vi "CVT1IndexReadTest.vi"() -> (3 "Unit Test Framework Results":T1)   [LabVIEW 2013, in "UnitTests.lvlib"]
uses:
  UnitTests.lvlib
  <vilib>/utf/common/utf_test_result_troll.ctl
  <vilib>/utf/common/utf_test_result.ctl
  <vilib>/utf/common/utf_test_result_failure.ctl
  <vilib>/utf/common/utf_test_comparison_operators.ctl
  <vilib>/utf/common/utf_vi_tag.ctl
  <vilib>/NI/Current Value Table/Read Index.vi
  <vilib>/NI/Current Value Table/DataTypes/I32_Read Index.vi
  <vilib>/NI/Current Value Table/Compatibility/TagConverter.vi
  <vilib>/NI/Current Value Table/Create Tags.vi
  <vilib>/NI/Current Value Table/Memory Block.vi
  <vilib>/NI/Current Value Table/DataTypes/I32_Memory Block.vi
  <vilib>/utf/NI_UnitTestFramework.lvlib
panel:
  out "Value":i32
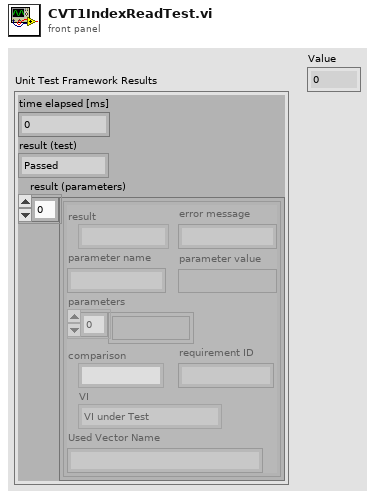
[diagram p1: front panel]
types:
  T1 = typedef "NI_UnitTestFramework.lvlib/utf_test_result_troll.ctl" = cluster{"time elapsed [ms]":u32, "result (test)":T2, "result (parameters)":T3[]}
  T2 = typedef "NI_UnitTestFramework.lvlib/utf_test_result.ctl" = enum16{"Passed", "Failed", "Error", "Skipped", "Not Processed"}
  T3 = typedef "NI_UnitTestFramework.lvlib/utf_test_result_failure.ctl" = cluster{"result":T2, "error message":string, "parameter name":string, "parameter value":variant, "parameters":variant[], "comparison":T4, "requirement ID":string, "VI":T5, "Used Vector Name":string}
  T4 = typedef "NI_UnitTestFramework.lvlib/utf_test_comparison_operators.ctl" = enum16{"=", "!=", ">", ">=", "<", "<=", "range", "symmetric tolerance", "asymmetric tolerance", "string contains", "string not contain", "array size", "string length", "array range", "by element", "array range (limit array)", "user-defined", "array contains", "array not contain", "vector length", "= (elm)", "!= (elm)", "= (case insensitive)", "!= (case insensitive)"}
  T5 = typedef "NI_UnitTestFramework.lvlib/utf_vi_tag.ctl" = enum16{"Setup VI", "VI under Test", "Teardown VI"}
  T6 = typedef "cvt_Tag Configuration.ctl" = cluster{"Name":string, "Data Type":T7, "Array":bool, "Size":u32, "Default":string, "Enum":string[], "Description":string}
  T7 = typedef "cvt_Data Types.ctl" = enum16{"Bool", "U8", "I32", "Double", "String", "Enum"}
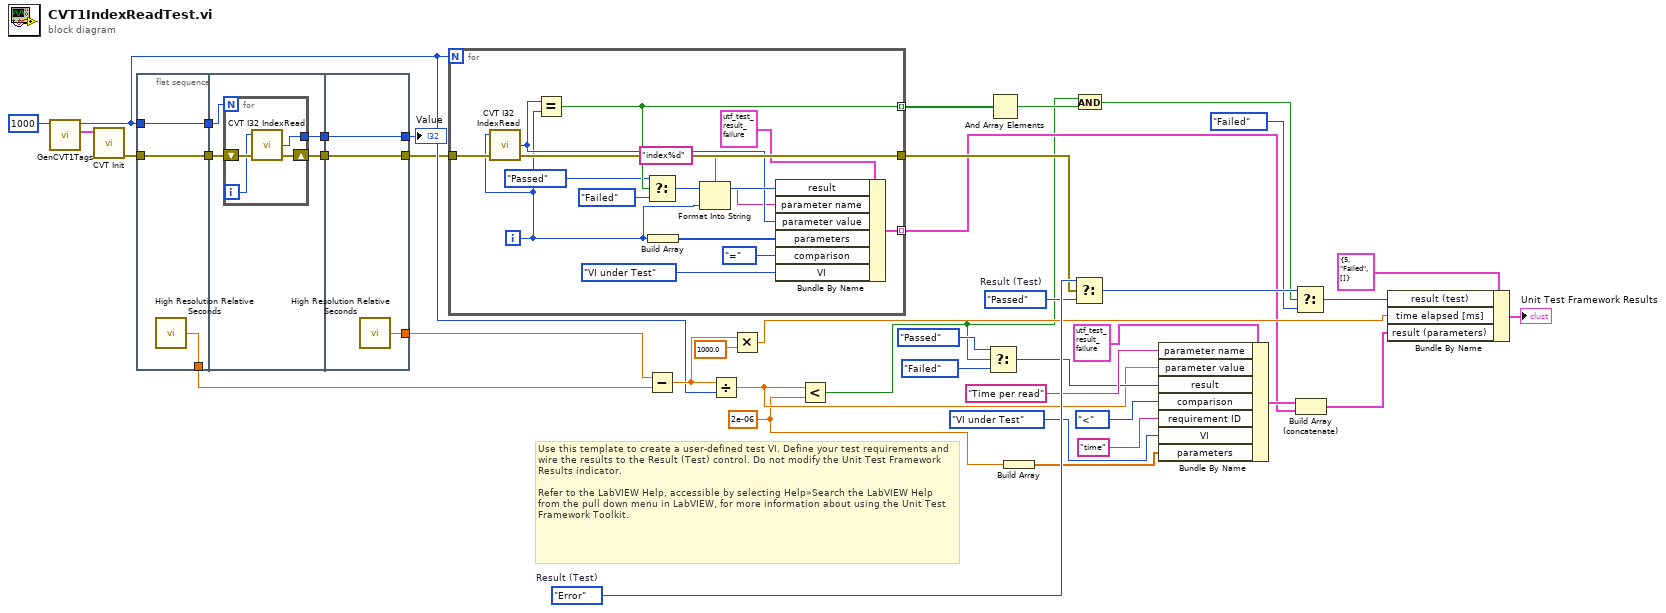
[diagram p0: block diagram]
diagram:
  w8 = 2e-06 ("y")
  w36 = utf_test_result."Error"  # Result (Test)
  w35 = utf_test_result."Passed"  # Result (Test)
  # "Use this template to create a user-defined test VI. Define your test requirements and wire the results to the Result (Test) control. Do not modify the Unit Test Framework Results indicator. \n\nRefer to the LabVIEW Help, accessible by selecting Help»Search the LabVIEW Help from the pull down menu in LabVIEW, for more information about using the Unit Test Framework Toolkit."
  n1 = call "GenCVT1Tags.vi"("Number of Tags in"=1000) -> ("Tags"=w1:T6[], "Number of Tags out"=w23:i32)  [unwired: 8 in, 1 out]
  n2 = call <vilib>:"CVT Init.vi"("Tag List"=w1) -> ("error out"=w29:errorcluster)  [unwired: 10 in]
  n3 = flat-sequence {
    tunnel: [w44] -> w38
    tunnel: w29 -> [w42]
    tunnel: [w43] -> w28
    tunnel: w23 -> [w43]
    tunnel: [w42] -> w27
    tunnel: w28 -> [w48]
    tunnel: w27 -> [w47]
    tunnel: [w46] -> w26
    tunnel: [w45] -> w3
    tunnel: [w55] -> w39
    tunnel: w26 -> [w54]
    tunnel: [w54] -> w22
    tunnel: [w53] -> w2
    tunnel: w3 -> [w53]
    frame #0 {
      n4 = call <vilib>:"High Resolution Relative Seconds.vi"() -> ("relative seconds"=w44:dbl)
    }
    frame #1 {
      n5 = for {
        N: w48 -> [_]
        shift-right: [w51] -> w46
        shift-left: w47 -> [w52]
        tunnel: [w50] -> w45
        i -> [w49]
        n6 = call <vilib>:"CVT I32 IndexRead.vi"("error in (no error)"=w52, "Tag Index"=w49) -> ("error out"=w51:errorcluster, "Value"=w50:i32)  [unwired: 2 in]
      }
    }
    frame #2 {
      n7 = call <vilib>:"High Resolution Relative Seconds.vi"() -> ("relative seconds"=w55:dbl)
    }
  }
  n8 = for {
    N: w23 -> [_]
    tunnel: w22 -> [w70]
    tunnel: [w69] -> w21
    tunnel: [w66] -> w20 mode=indexing
    tunnel: [w62] -> w6 mode=indexing
    i -> [w58]
    n9 = call <vilib>:"CVT I32 IndexRead.vi"("error in (no error)"=w70, "Tag Index"=w58) -> ("error out"=w69:errorcluster, "Value"=w59:i32)  [unwired: 2 in]
    n10 = Equal?(x=w59, y=w58) -> (x = y?=w66:bool)
    n11 = Select(t=utf_test_result."Passed" ("result"), s=w66, f=utf_test_result."Failed" ("result")) -> (s? t:f=w63:T2)
    n12 = Build Array(w58) -> (w60:i32[])
    n13 = Format Into String(format string="index%d", w58) -> (resulting string=w57:string)  [unwired: 2 in, 1 out]
    n14 = Bundle By Name(cluster=T3 {"result"=enum."Passed", "error message"="", "parameter name"="", "parameter value"=variant, "parameters"=[], "comparison"=enum."=", "requirement ID"="", "VI"=enum."Setup VI", "Used Vector Name"=""} ("Unit Test Framework - result (parameters)"), "result"=w63, "parameter name"=w57, "parameter value"=w59, "parameters"=w60, "comparison"=utf_test_comparison_operators."=", "VI"=utf_vi_tag."VI under Test") -> (w62:T3)
  }
  n15 = Subtract(x=w39, y=w38) -> (x-y=w25:dbl)
  n16 = Divide(x=w25, y=w23) -> (x/y=w11:dbl)
  n17 = Multiply(x=w25, y=1000.0) -> (x*y=w30:dbl)
  n18 = Less?(x=w11, y=w8) -> (x < y?=w4:bool)
  n19 = Select(t=utf_test_result."Passed" ("result"), s=w4, f=utf_test_result."Failed" ("result")) -> (s? t:f=w12:T2)
  n20 = And Array Elements(Boolean array=w20) -> (logical AND=w19:bool)
  n21 = Build Array(w8) -> (w7:dbl[])
  n22 = Select(t=w36, s=w21, f=w35) -> (s? t:f=w18:T2)
  n23 = And(x=w4, y=w19) -> (x .and. y?=w5:bool)
  n24 = Bundle By Name(cluster=T3 {"result"=enum."Passed", "error message"="", "parameter name"="", "parameter value"=variant, "parameters"=[], "comparison"=enum."=", "requirement ID"="", "VI"=enum."Setup VI", "Used Vector Name"=""} ("Unit Test Framework - result (parameters)"), "parameter name"="Time per read", "parameter value"=w11, "result"=w12, "comparison"=utf_test_comparison_operators."<", "requirement ID"="time", "VI"=utf_vi_tag."VI under Test", "parameters"=w7) -> (w33:T3)
  n25 = Select(t=w18, s=w5, f=utf_test_result."Failed") -> (s? t:f=w16:T2)
  n26 = Build Array (concatenate)(w33, w6) -> (w32:T3[])
  n27 = Bundle By Name(cluster=T1 {"time elapsed [ms]"=5, "result (test)"=enum."Failed", "result (parameters)"=[]} ("Unit Test Framework - Result"), "result (test)"=w16, "time elapsed [ms]"=w30, "result (parameters)"=w32) -> (→"Unit Test Framework Results":T1)
  "Value" <- w2
